vi "main.vi"() -> ()   [LabVIEW 2017]
uses:
  <vilib>/userdefined/High Color/IMAQdx.ctl
  <vilib>/vision/driver/NI_Vision_Acquisition_Software.lvlib
  <vilib>/vision/NI_Vision_Development_Module.lvlib
panel:
  in  "Left":bool
  in  "Right":bool
  in  "Save":bool
  out "People":i32 caption="Numeric"
  out "Image":T1(plugin-control)
  in  "Stop":bool
  in  "Session In":T2
  # "People detected:"
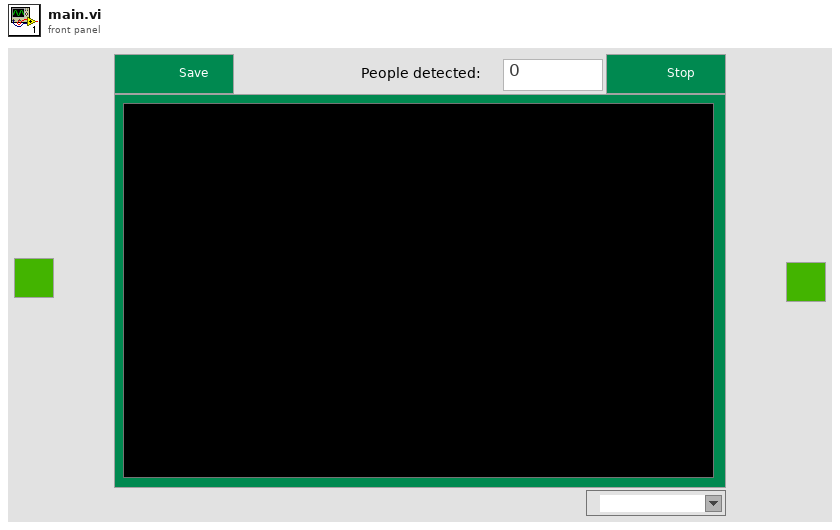
[diagram p1: front panel]
types:
  T1 = typedef "IMAQ Image.ctl" = refnum<image>
  T2 = typedef "IMAQdx.ctl" = refnum<k21>
  T3 = typedef "Image Type" = u32
  T4 = typedef "IMAQ Rectangle" = cluster{"Left":i32, "Top":i32, "Right":i32, "Bottom":i32, "Rotation":dbl}
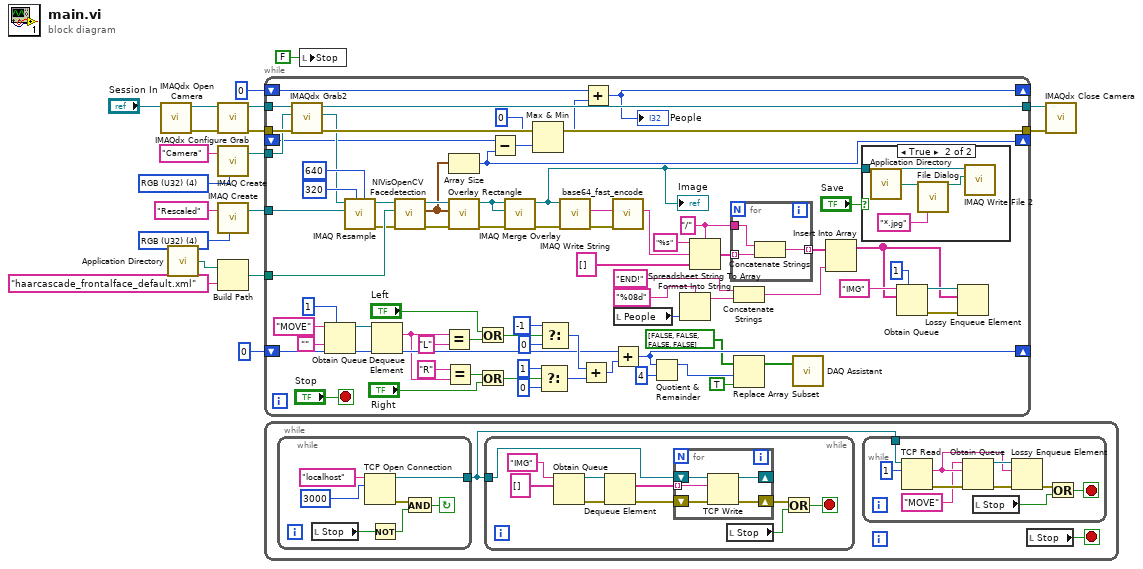
[diagram p0: block diagram]
diagram:
  w5 = T3 4 items=["Grayscale (U8)", "Grayscale (I16)", "Grayscale (SGL)", "Complex (CSG)", "RGB (U32)", "HSL (U32)", "RGB (U64)", "Grayscale (U16)"] ("Image Type")
  w11 = T3 4 items=["Grayscale (U8)", "Grayscale (I16)", "Grayscale (SGL)", "Complex (CSG)", "RGB (U32)", "HSL (U32)", "RGB (U64)", "Grayscale (U16)"] ("Image Type")
  n1 = call <vilib>:"IMAQdx Open Camera.vi"("Session In"="Session In") -> ("error out"=w16:errorcluster, "Session Out"=w19:T2)  [unwired: 9 in]
  n2 = call <vilib>:"Application Directory.vi"() -> ("Application Directory"=w9:path)
  n3 = call <vilib>:"IMAQdx Configure Grab.vi"("error in"=w16, "Session In"=w19) -> ("error out"=w15:errorcluster, "Session Out"=w18:T2)  [unwired: 8 in]
  n4 = call "IMAQ Create"("Image Name"="Camera", "Image Type"=w11) -> ("New Image"=w10:T1)  [unwired: 3 in, 1 out]
  n5 = call "IMAQ Create"("Image Name"="Rescaled", "Image Type"=w5) -> ("New Image"=w4:T1)  [unwired: 3 in, 1 out]
  n6 = Build Path(base path=w9, name or relative path="haarcascade_frontalface_default.xml") -> (appended path=w7:path)
  n7 = while {
    tunnel: w18 -> [w93]
    tunnel: [w92] -> w17
    tunnel: w15 -> [w91]
    tunnel: [w90] -> w14
    tunnel: w10 -> [w89]
    tunnel: w7 -> [w76]
    tunnel: w4 -> [w81]
    shift-right: [w31] -> _
    shift-left: 0 -> [w57]
    shift-right: [w24] -> _
    shift-left: _ -> [w29]
    shift-right: [w23] -> _
    shift-left: 0 -> [w25]
    stop <- "Stop" stop-if-true
    w83 = "/" ("delimiter (Tab)")
    n8 = call <vilib>:"IMAQdx Grab2.vi"("error in"=w91, "Image In"=w89, "Session In"=w93) -> ("error out"=w90:errorcluster, "Image Out"=w72:T1, "Session Out"=w92:T2)  [unwired: 5 in, 1 out]
    n9 = Obtain Queue(max queue size (-1, unlimited)=1, name (unnamed)="MOVE", element data type="") -> (queue out=w52:refnum<queue>, error out=w49:errorcluster)  [unwired: 2 in, 1 out]
    n10 = call "IMAQ Resample"("X Resolution"=640, "Y Resolution"=320, "Image Dst"=w81, "Image Src"=w72) -> ("error out"=w75:errorcluster, "Image Dst Out"=w77:T1)  [unwired: 6 in]
    n11 = Dequeue Element(queue=w52, error in (no error)=w49) -> (element=w48:string)  [unwired: 1 in, 3 out]
    n12 = call <vilib>:"NIVisOpenCV Facedetection.vi"("error in (no error)"=w75, "Face Cascade Path"=w76, "Image Src"=w77) -> ("error out"=w74:errorcluster, "Faces"=w67:T4[], "Image Dst Out"=w78:T1)  [unwired: 5 in, 1 out]
    n13 = Equal?(x=w48, y="L" ("delimiter (Tab)")) -> (x = y?=w44:bool)
    n14 = Equal?(x="R" ("delimiter (Tab)"), y=w48) -> (x = y?=w41:bool)
    n15 = Array Size(array=w67) -> (size(s)=w24:i32)
    n16 = call "Overlay Rectangle.vi"("error in (no error)"=w74, "Faces"=w67, "Image in"=w78) -> ("error out"=w69:errorcluster, "Image out"=w70:T1)  [unwired: 7 in]
    n17 = Or(x="Left", y=w44) -> (x .or. y?=w40:bool)
    n18 = Or(x=w41, y="Right") -> (x .or. y?=w43:bool)
    n19 = Subtract(x=w29, y=w24) -> (x-y=w28:i32)
    n20 = call "IMAQ Merge Overlay"("error in (no error)"=w69, "Image Dst"=w70, "Image Src"=w70) -> ("error out"=w68:errorcluster, "Image Dst Out"=w65:T1)  [unwired: 7 in]
    "Image" <- w65
    n21 = Max & Min(x=0, y=w28) -> (max(x,y)=w26:i32)  [unwired: 1 out]
    n22 = Select(t=1, s=w43, f=0) -> (s? t:f=w59:i32)
    n23 = Select(t=-1, s=w40, f=0) -> (s? t:f=w60:i32)
    n24 = call-poly "IMAQ Write String"("error in (no error)"=w68, "Image"=w65) -> ("error out"=w73:errorcluster, "FileString"=w88:string)  [unwired: 7 in, 1 out]
    n25 = Add(x=w60, y=w59) -> (x+y=w58:i32)
    n26 = Add(x=w25, y=w26) -> (x+y=w23:i32)
    "People" <- w23
    n27 = call "base64_fast_encode.vi"("error in (no error)"=w73, "string in (not encoded)"=w88) -> ("string out (base64-encoded)"=w86:string)  [unwired: 8 in, 1 out]
    n28 = Add(x=w57, y=w58) -> (x+y=w31:i32)
    n29 = local read "People"() -> (w35:i32)
    n30 = Quotient & Remainder(x=w31, y=4) -> (x-y*floor(x/y)=w22:i32)  [unwired: 1 out]
    n31 = Format Into String(format string="%08d", w35) -> (resulting string=w37:string)  [unwired: 2 in, 1 out]
    n32 = Spreadsheet String To Array(delimiter (Tab)=w83, format string="%s", spreadsheet string=w86, array type (2D Dbl)=string[] []) -> (array=w84:string[])
    n33 = for {
      tunnel: w84 -> [w100] mode=indexing
      tunnel: w83 -> [w99]
      tunnel: [w98] -> w82 mode=indexing
      n34 = Concatenate Strings(w99, w100) -> (w98:string)
    }
    n35 = Concatenate Strings("END!" ("new element/subarray"), w37) -> (w38:string)
    n36 = Replace Array Subset(array=bool[] [FALSE, FALSE, FALSE, FALSE], new element=TRUE ("new element/subarray"), index=w22) -> (w20:bool[])
    n37 = call "DAQ Assistant"("data"=w20) -> ()  [unwired: 17 in, 2 out]
    n38 = Insert Into Array(array=w82, new element=w38) -> (w53:string[])  [unwired: 1 in]
    n39 = case shown="True" "Save" {
      tunnel: w65 -> [_ w97]
      frame False {
      }
      frame True {
        n40 = call <vilib>:"Application Directory.vi"() -> ("Application Directory"=w95:path)
        n41 = call "File Dialog"("start path"=w95, "pattern (all files)"="*.jpg") -> ("selected path"=w96:path)  [unwired: 10 in, 3 out]
        n42 = call-poly "IMAQ Write File 2"("File Path"=w96, "Image"=w97) -> ()  [unwired: 8 in, 2 out]
      }
    }
    n43 = Obtain Queue(max queue size (-1, unlimited)=1, name (unnamed)="IMG", element data type=w53) -> (queue out=w54:refnum<queue>, error out=w36:errorcluster)  [unwired: 2 in, 1 out]
    n44 = Lossy Enqueue Element(queue=w54, element=w53, error in (no error)=w36) -> ()  [unwired: 4 out]
  }
  n45 = while {
    stop <- w102 stop-if-true
    n46 = while {
      tunnel: [w132] -> w101
      stop <- w130 continue-if-true
      n47 = local read "Stop"() -> (w128:bool)
      n48 = TCP Open Connection(address="localhost", remote port or service name=u16 3000) -> (connection ID=w132:refnum<k5>, error out=w131:errorcluster)  [unwired: 3 in]
      n49 = Not(x=w128) -> (.not. x?=w129:bool)
      n50 = And(x=w131, y=w129) -> (x .and. y?=w130:bool)
    }
    n51 = while {
      tunnel: w101 -> [w113]
      stop <- w114 stop-if-true
      n52 = Obtain Queue(name (unnamed)="IMG", element data type=string[] [] ("array type (2D Dbl)")) -> (queue out=w121:refnum<queue>, error out=w118:errorcluster)  [unwired: 3 in, 1 out]
      n53 = Dequeue Element(queue=w121, error in (no error)=w118) -> (element=w120:string[], error out=w119:errorcluster)  [unwired: 1 in, 2 out]
      n54 = for {
        shift-right: [w125] -> _
        shift-left: w113 -> [w127]
        shift-right: [w124] -> w116
        shift-left: w119 -> [w126]
        tunnel: w120 -> [w123] mode=indexing
        n55 = TCP Write(connection ID=w127, data in=w123, error in (no error)=w126) -> (connection ID out=w125:refnum<k5>, error out=w124:errorcluster)  [unwired: 1 in, 1 out]
      }
      n56 = local read "Stop"() -> (w115:bool)
      n57 = Or(x=w116, y=w115) -> (x .or. y?=w114:bool)
    }
    n58 = while {
      tunnel: w101 -> [w111]
      stop <- w109 stop-if-true
      n59 = TCP Read(connection ID=w111, bytes to read=1) -> (data out=w105:string, error out=w108:errorcluster)  [unwired: 3 in, 1 out]
      n60 = Obtain Queue(name (unnamed)="MOVE", element data type=w105, error in (no error)=w108) -> (queue out=w107:refnum<queue>, error out=w106:errorcluster)  [unwired: 2 in, 1 out]
      n61 = local read "Stop"() -> (w110:bool)
      n62 = Lossy Enqueue Element(queue=w107, element=w105, error in (no error)=w106) -> (error out=w103:errorcluster)  [unwired: 3 out]
      n63 = Or(x=w103, y=w110) -> (x .or. y?=w109:bool)
    }
    n64 = local read "Stop"() -> (w102:bool)
  }
  n65 = local write "Stop"(FALSE ("Stop")) -> ()
  n66 = call <vilib>:"IMAQdx Close Camera.vi"("error in"=w14, "Session In"=w17) -> ()  [unwired: 9 in, 1 out]
